vi "MegaAnalysis5.vi"() -> ()   [LabVIEW 2016] (continued)
                          frame #4 {
                            n844 = Array Size(array=w2082) -> (size(s)=w2081:i32)
                            n845 = Divide(x=w2081, y=2) -> (x/y=w2079:dbl)
                            n846 = for {
                              N: w2079 -> [_]
                              tunnel: w2078 -> [w2087]
                              tunnel: w2077 -> [w2084]
                              tunnel: w2076 -> [w2083]
                              i -> [w2088]
                              n847 = Multiply(x=2, y=w2088) -> (x*y=w2091:i32)
                              n848 = Increment(x=w2091) -> (x+1=w2090:i32)
                              n849 = call "readbinary.vi"(7:w2084, "base path"=w2087, "file index"=w2090, "data column"="bdot") -> ("data"=w2086:ext[])  [unwired: 7 out]
                              n850 = call "writebinary.vi"(7:w2083, "base path"=w2087, "file index"=w2088, "data column"="bdtt", "data"=w2086) -> ()  [unwired: 7 out]
                            }
                          }
                          frame #5 {
                            n851 = Array Size(array=w2099) -> (size(s)=w2098:i32)
                            n852 = Divide(x=w2098, y=2) -> (x/y=w2096:dbl)
                            n853 = for {
                              N: w2096 -> [_]
                              tunnel: w2095 -> [w2104]
                              tunnel: w2094 -> [w2101]
                              tunnel: w2093 -> [w2100]
                              i -> [w2105]
                              n854 = Multiply(x=2, y=w2105) -> (x*y=w2107:i32)
                              n855 = Increment(x=w2107) -> ()  [unwired: 1 out]
                              n856 = call "readbinary.vi"(7:w2101, "base path"=w2104, "file index"=w2107, "data column"="indx") -> ("data"=w2103:ext[])  [unwired: 7 out]
                              n857 = call "writebinary.vi"(7:w2100, "base path"=w2104, "file index"=w2105, "data column"="indt", "data"=w2103) -> ()  [unwired: 7 out]
                            }
                          }
                          frame #6 {
                            n858 = Array Size(array=w2115) -> (size(s)=w2114:i32)
                            n859 = Divide(x=w2114, y=2) -> (x/y=w2112:dbl)
                            n860 = for {
                              N: w2112 -> [_]
                              tunnel: w2111 -> [w2120]
                              tunnel: w2110 -> [w2117]
                              tunnel: w2109 -> [w2116]
                              i -> [w2121]
                              n861 = Multiply(x=2, y=w2121) -> (x*y=w2123:i32)
                              n862 = Increment(x=w2123) -> ()  [unwired: 1 out]
                              n863 = call "readbinary.vi"(7:w2117, "base path"=w2120, "file index"=w2123, "data column"="time") -> ("data"=w2119:ext[])  [unwired: 7 out]
                              n864 = call "writebinary.vi"(7:w2116, "base path"=w2120, "file index"=w2121, "data column"="timt", "data"=w2119) -> ()  [unwired: 7 out]
                            }
                          }
                          frame #7 {
                            n865 = Array Size(array=w2136) -> (size(s)=w2139:i32)
                            n866 = Divide(x=w2139, y=2) -> (x/y=w2137:dbl)
                            n867 = for {
                              N: w2137 -> [_]
                              tunnel: w2125 -> [_]
                              tunnel: w2136 -> [w2148]
                              tunnel: w2135 -> [w2147]
                              tunnel: w2134 -> [w2144]
                              tunnel: [w2143] -> w2127 mode=indexing
                              tunnel: w2133 -> [w2142]
                              tunnel: [w2140] -> w2128 mode=indexing
                              i -> [w2150]
                              n868 = Multiply(x=2, y=w2150) -> (x*y=w2141:i32)
                              n869 = Index Array(array=w2148, index=w2141) -> (element=w2146:string)
                              n870 = Increment(x=w2141) -> (x+1=w2149:i32)
                              n871 = Index Array(array=w2148, index=w2149) -> (element=w2145:string)
                              n872 = case shown="1" w2147 {
                                tunnel: w2146 -> [_ w2158]
                                tunnel: w2145 -> [w2152 w2157]
                                tunnel: [w2152 w2155] -> w2143
                                tunnel: w2144 -> [_ w2156]
                                frame 0, Default {
                                }
                                frame 1 {
                                n873 = String Subset(string=w2158, length (rest)=w2156) -> (substring=w2154:string)  [unwired: 1 out]
                                n874 = String Subset(string=w2157, length (rest)=w2156) -> (substring=w2153:string)  [unwired: 1 out]
                                n875 = Concatenate Strings(w2153, w2154) -> (w2155:string)
                                }
                              }
                              n876 = Index Array(array=w2142, index=w2141) -> (element=w2140:path)
                            }
                            n877 = Build Path(base path=w2125, name or relative path="files2") -> (appended path=w2131:path)
                            n878 = call-poly <vilib>:"Write To Spreadsheet File.vi"("1D data"=w2127, "file path (dialog if empty)"=w2131) -> ()  [unwired: 4 in, 3 out]
                            n879 = Build Path(base path=w2125, name or relative path="paths2") -> (appended path=w2129:path)
                            n880 = Path To String(path=w2128) -> (string=w2126:string[])
                            n881 = call-poly <vilib>:"Write To Spreadsheet File.vi"("1D data"=w2126, "file path (dialog if empty)"=w2129) -> ()  [unwired: 4 in, 3 out]
                          }
                        }
                      }
                    }
                  }
                }
                n882 = global write "status.vi" "String"("selecting data") -> ()
              }
            }
          }
          frame #2 {
            n883 = case shown="True" "?" {
              tunnel: w2162 -> [_ w2167]
              tunnel: w2161 -> [_ w2166]
              tunnel: w2160 -> [_ w2165]
              tunnel: w2159 -> [_ w2164]
              frame False {
              }
              frame True {
                n884 = case shown="True" w2165 {
                  tunnel: w2167 -> [_ w2170]
                  tunnel: w2166 -> [_ w2169]
                  tunnel: w2164 -> [_ w2168]
                  frame False {
                  }
                  frame True {
                    n885 = stacked-sequence {
                      seq-local: [w2181 _] -> [_ w2212]
                      seq-local: [w2182 _] -> [_ w2215]
                      seq-local: [w2173 _] -> [_ w2206]
                      seq-local: [w2172 _] -> [_ w2204]
                      tunnel: w2170 -> [w2177 _]
                      tunnel: w2169 -> [w2180 _]
                      tunnel: w2168 -> [w2171 _]
                      frame #0 {
                        n886 = Build Path(base path=w2177, name or relative path="paths2") -> (appended path=w2172:path)
                        n887 = Build Path(base path=w2177, name or relative path="files2") -> (appended path=w2173:path)
                        n888 = call "readbinary.vi"(7:w2171, "base path"=w2177, "file index"=0, "data column"="indt") -> ("data"=w2176:ext[])  [unwired: 7 out]
                        n889 = call-poly <vilib>:"Read From Spreadsheet File.vi"("file path (dialog if empty)"=w2172) -> ("first row"=w2183:string[])  [unwired: 3 in, 7 out]
                        n890 = Array Size(array=w2176) -> (size(s)=w2175:i32)
                        n891 = for {
                          N: w2175 -> [_]
                          tunnel: [0] -> w2174 mode=indexing
                        }
                        n892 = call-poly <vilib>:"Read From Spreadsheet File.vi"("file path (dialog if empty)"=w2173) -> ("first row"=w2181:string[])  [unwired: 3 in, 7 out]
                        n893 = String To Path(string=w2183) -> (path=w2182:path[])
                        n894 = for {
                          tunnel: w2181 -> [w2194]
                          tunnel: w2180 -> [w2191] mode=indexing
                          tunnel: w2177 -> [w2190]
                          tunnel: w2174 -> [w2195]
                          tunnel: w2171 -> [w2187]
                          n895 = Array Size(array=w2194) -> (size(s)=w2189:i32)
                          n896 = for {
                            N: w2189 -> [_]
                            tunnel: w2194 -> [_] mode=indexing
                            tunnel: w2190 -> [w2202]
                            shift-right: [w2201] -> w2193
                            shift-left: w2195 -> [w2199]
                            tunnel: w2191 -> [w2198]
                            tunnel: w2187 -> [w2196]
                            i -> [w2197]
                            n897 = call "readbinary.vi"(7:w2196, "base path"=w2202, "file index"=w2197, "data column"=w2198) -> ("data"=w2200:ext[])  [unwired: 7 out]
                            n898 = Add(x=w2200, y=w2199) -> (x+y=w2201:ext[])
                          }
                          n899 = Divide(x=w2193, y=w2189) -> (x/y=w2192:ext[])
                          n900 = call "writebinary.vi"(7:w2187, "base path"=w2190, "file index"=0, "data column"=w2191, "data"=w2192) -> ()  [unwired: 7 out]
                        }
                      }
                      frame #1 {
                        n901 = Index Array(array=w2215, index=0) -> (element=w2209:path)
                        n902 = case shown="True" "?" {
                          tunnel: w2212 -> [w2219 w2223]
                          tunnel: "append string onto file name" -> [w2218 w2224]
                          tunnel: "?" -> [_ w2222]
                          tunnel: [w2216 w2221] -> w2208
                          frame False {
                            n903 = Index Array(array=w2219, index=0) -> (element=w2217:string)
                            n904 = Concatenate Strings(w2218, w2217) -> (w2216:string)
                          }
                          frame True {
                            n905 = for {
                              shift-right: [w2225] -> w2221
                              shift-left: w2224 -> [w2227]
                              tunnel: w2223 -> [w2230] mode=indexing
                              tunnel: w2222 -> [w2228]
                              n906 = String Subset(string=w2230, offset (0)=0, length (rest)=w2228) -> (substring=w2226:string)
                              n907 = Concatenate Strings(w2227, w2226) -> (w2225:string)
                            }
                          }
                        }
                        n908 = Build Array(w2209) -> (w2207:path[])
                        n909 = Path To String(path=w2207) -> (string=w2203:string[])
                        n910 = Build Array(w2208) -> (w2205:string[])
                        n911 = call-poly <vilib>:"Write To Spreadsheet File.vi"("1D data"=w2205, "file path (dialog if empty)"=w2206) -> ()  [unwired: 4 in, 3 out]
                        n912 = call-poly <vilib>:"Write To Spreadsheet File.vi"("1D data"=w2203, "file path (dialog if empty)"=w2204) -> ()  [unwired: 4 in, 3 out]
                      }
                    }
                  }
                }
              }
            }
          }
          frame #3 {
            n913 = case shown="False" w2233 {
              tunnel: w2232 -> [_ w2235]
              tunnel: w2231 -> [_ w2234]
              frame False {
              }
              frame True {
                n914 = stacked-sequence {
                  seq-local: [w2236 _ _ _ _ _ _] -> [_ w2242 w2300 w2318 w2336 w2354 w2373]
                  tunnel: w2235 -> [w2239 w2243 w2301 w2319 w2337 w2355 w2374]
                  tunnel: [w2236 _ _ _ _ _ _] -> _
                  tunnel: w2234 -> [_ w2241 w2299 w2317 w2335 w2353 w2372]
                  frame #0 {
                    n915 = Build Path(base path=w2239, name or relative path="files2") -> (appended path=w2238:path)
                    n916 = call-poly <vilib>:"Read From Spreadsheet File.vi"("format (%s)"="%s", "file path (dialog if empty)"=w2238) -> ("first row"=w2236:string[])  [unwired: 2 in, 7 out]
                  }
                  frame #1 {
                    n917 = case shown="0, Default" "data options" {
                      tunnel: w2243 -> [w2247 w2256 w2265 w2277 w2289]
                      tunnel: w2242 -> [w2246 w2255 w2264 w2276 w2288]
                      tunnel: w2241 -> [w2245 w2254 w2263 w2275 w2287]
                      frame 0, Default {
                        n918 = for {
                          tunnel: w2247 -> [w2249]
                          tunnel: w2246 -> [_] mode=indexing
                          tunnel: w2245 -> [w2248]
                          i -> [w2250]
                          n919 = call "readbinary.vi"(7:w2248, "base path"=w2249, "file index"=w2250, "data column"="dt1t") -> ("data"=w2252:ext[])  [unwired: 7 out]
                          n920 = call "writebinary.vi"(7:w2248, "base path"=w2249, "file index"=w2250, "data column"="dt1t", "data"=w2252) -> ()  [unwired: 7 out]
                        }
                      }
                      frame 1 {
                        n921 = for {
                          tunnel: w2256 -> [w2258]
                          tunnel: w2255 -> [_] mode=indexing
                          tunnel: w2254 -> [w2257]
                          i -> [w2259]
                          n922 = call "readbinary.vi"(7:w2257, "base path"=w2258, "file index"=w2259, "data column"="dt2t") -> ("data"=w2261:ext[])  [unwired: 7 out]
                          n923 = call "writebinary.vi"(7:w2257, "base path"=w2258, "file index"=w2259, "data column"="dt1t", "data"=w2261) -> ()  [unwired: 7 out]
                        }
                      }
                      frame 2 {
                        n924 = for {
                          tunnel: w2265 -> [w2270]
                          tunnel: w2264 -> [_] mode=indexing
                          tunnel: w2263 -> [w2266]
                          i -> [w2271]
                          n925 = call "readbinary.vi"(7:w2266, "base path"=w2270, "file index"=w2271, "data column"="dt2t") -> ("data"=w2268:ext[])  [unwired: 7 out]
                          n926 = call "readbinary.vi"(7:w2266, "base path"=w2270, "file index"=w2271, "data column"="dt1t") -> ("data"=w2269:ext[])  [unwired: 7 out]
                          n927 = Subtract(x=w2269, y=w2268) -> (x-y=w2267:ext[])
                          n928 = call "writebinary.vi"(7:w2266, "base path"=w2270, "file index"=w2271, "data column"="dt1t", "data"=w2267) -> ()  [unwired: 7 out]
                        }
                      }
                      frame 3 {
                        n929 = for {
                          tunnel: w2277 -> [w2282]
                          tunnel: w2276 -> [_] mode=indexing
                          tunnel: w2275 -> [w2278]
                          i -> [w2283]
                          n930 = call "readbinary.vi"(7:w2278, "base path"=w2282, "file index"=w2283, "data column"="dt2t") -> ("data"=w2280:ext[])  [unwired: 7 out]
                          n931 = call "readbinary.vi"(7:w2278, "base path"=w2282, "file index"=w2283, "data column"="dt1t") -> ("data"=w2281:ext[])  [unwired: 7 out]
                          n932 = Add(x=w2281, y=w2280) -> (x+y=w2279:ext[])
                          n933 = call "writebinary.vi"(7:w2278, "base path"=w2282, "file index"=w2283, "data column"="dt1t", "data"=w2279) -> ()  [unwired: 7 out]
                        }
                      }
                      frame 4 {
                        n934 = for {
                          tunnel: w2289 -> [w2294]
                          tunnel: w2288 -> [_] mode=indexing
                          tunnel: w2287 -> [w2290]
                          i -> [w2295]
                          n935 = call "readbinary.vi"(7:w2290, "base path"=w2294, "file index"=w2295, "data column"="dt2t") -> ("data"=w2292:ext[])  [unwired: 7 out]
                          n936 = call "readbinary.vi"(7:w2290, "base path"=w2294, "file index"=w2295, "data column"="dt1t") -> ("data"=w2293:ext[])  [unwired: 7 out]
                          n937 = Re/Im To Polar(2:w2293, 3:w2292) -> (1:w2291:ext[])  [unwired: 1 out]
                          n938 = call "writebinary.vi"(7:w2290, "base path"=w2294, "file index"=w2295, "data column"="dt1t", "data"=w2291) -> ()  [unwired: 7 out]
                        }
                      }
                    }
                  }
                  frame #2 {
                    n939 = case shown="True" "?" {
                      tunnel: w2301 -> [_ w2305]
                      tunnel: w2300 -> [_ w2304]
                      tunnel: w2299 -> [_ w2303]
                      frame False {
                      }
                      frame True {
                        n940 = for {
                          tunnel: w2305 -> [w2312]
                          tunnel: w2304 -> [_] mode=indexing
                          tunnel: w2303 -> [w2306]
                          i -> [w2313]
                          n941 = call "readbinary.vi"(7:w2306, "base path"=w2312, "file index"=w2313, "data column"="dt1t") -> ("data"=w2308:ext[])  [unwired: 7 out]
                          n942 = call "readbinary.vi"(7:w2306, "base path"=w2312, "file index"=w2313, "data column"="timt") -> ("data"=w2311:ext[])  [unwired: 7 out]
                          n943 = Multiply(x="?", y=w2311) -> (x*y=w2309:ext[])
                          n944 = Add(x=w2308, y=w2309) -> (x+y=w2307:ext[])
                          n945 = call "writebinary.vi"(7:w2306, "base path"=w2312, "file index"=w2313, "data column"="dt1t", "data"=w2307) -> ()  [unwired: 7 out]
                        }
                      }
                    }
                  }
                  frame #3 {
                    n946 = case shown="True" "?" {
                      tunnel: w2319 -> [_ w2323]
                      tunnel: w2318 -> [_ w2322]
                      tunnel: w2317 -> [_ w2321]
                      frame False {
                      }
                      frame True {
                        n947 = for {
                          tunnel: w2323 -> [w2330]
                          tunnel: w2322 -> [_] mode=indexing
                          tunnel: w2321 -> [w2324]
                          i -> [w2331]
                          n948 = call "readbinary.vi"(7:w2324, "base path"=w2330, "file index"=w2331, "data column"="dt1t") -> ("data"=w2326:ext[])  [unwired: 7 out]
                          n949 = call "readbinary.vi"(7:w2324, "base path"=w2330, "file index"=w2331, "data column"="bdtt") -> ("data"=w2329:ext[])  [unwired: 7 out]
                          n950 = Multiply(x="?", y=w2329) -> (x*y=w2327:ext[])
                          n951 = Add(x=w2326, y=w2327) -> (x+y=w2325:ext[])
                          n952 = call "writebinary.vi"(7:w2324, "base path"=w2330, "file index"=w2331, "data column"="dt1t", "data"=w2325) -> ()  [unwired: 7 out]
                        }
                      }
                    }
                  }
                  frame #4 {
                    n953 = case shown="True" "?" {
                      tunnel: w2337 -> [_ w2341]
                      tunnel: w2336 -> [_ w2340]
                      tunnel: w2335 -> [_ w2339]
                      frame False {
                      }
                      frame True {
                        n954 = for {
                          tunnel: w2341 -> [w2348]
                          tunnel: w2340 -> [_] mode=indexing
                          tunnel: w2339 -> [w2342]
                          i -> [w2349]
                          n955 = call "readbinary.vi"(7:w2342, "base path"=w2348, "file index"=w2349, "data column"="dt1t") -> ("data"=w2344:ext[])  [unwired: 7 out]
                          n956 = call "readbinary.vi"(7:w2342, "base path"=w2348, "file index"=w2349, "data column"="bclt") -> ("data"=w2347:ext[])  [unwired: 7 out]
                          n957 = Multiply(x="?", y=w2347) -> (x*y=w2345:ext[])
                          n958 = Add(x=w2344, y=w2345) -> (x+y=w2343:ext[])
                          n959 = call "writebinary.vi"(7:w2342, "base path"=w2348, "file index"=w2349, "data column"="dt1t", "data"=w2343) -> ()  [unwired: 7 out]
                        }
                      }
                    }
                  }
                  frame #5 {
                    n960 = case shown="True" "?" {
                      tunnel: w2355 -> [_ w2359]
                      tunnel: w2354 -> [_ w2358]
                      tunnel: w2353 -> [_ w2357]
                      frame False {
                      }
                      frame True {
                        n961 = for {
                          tunnel: w2359 -> [w2367]
                          tunnel: [w2361] -> _ mode=indexing
                          tunnel: w2358 -> [w2361] mode=indexing
                          tunnel: w2357 -> [w2360]
                          i -> [w2368]
                          n962 = call "readbinary.vi"(7:w2360, "base path"=w2367, "file index"=w2368, "data column"="dt1t") -> ("data"=w2363:ext[])  [unwired: 7 out]
                          n963 = call "readbinary.vi"(7:w2360, "base path"=w2367, "file index"=w2368, "data column"="dt2t") -> ("data"=w2366:ext[])  [unwired: 7 out]
                          n964 = Multiply(x="?", y=w2366) -> (x*y=w2364:ext[])
                          n965 = Add(x=w2363, y=w2364) -> (x+y=w2362:ext[])
                          n966 = call "writebinary.vi"(7:w2360, "base path"=w2367, "file index"=w2368, "data column"="dt1t", "data"=w2362) -> ()  [unwired: 7 out]
                        }
                      }
                    }
                  }
                  frame #6 {
                    n967 = case shown="True" "?" {
                      tunnel: w2374 -> [_ w2378]
                      tunnel: w2373 -> [_ w2377]
                      tunnel: w2372 -> [_ w2376]
                      frame False {
                      }
                      frame True {
                        n968 = for {
                          tunnel: w2378 -> [w2383]
                          tunnel: w2377 -> [_] mode=indexing
                          tunnel: w2376 -> [w2379]
                          i -> [w2384]
                          n969 = call "readbinary.vi"(7:w2379, "base path"=w2383, "file index"=w2384, "data column"="dt1t") -> ("data"=w2381:ext[])  [unwired: 7 out]
                          n970 = Multiply(x="?", y=w2381) -> (x*y=w2380:ext[])
                          n971 = call "writebinary.vi"(7:w2379, "base path"=w2383, "file index"=w2384, "data column"="dt1t", "data"=w2380) -> ()  [unwired: 7 out]
                        }
                      }
                    }
                  }
                }
              }
            }
          }
          frame #4 {
            n972 = case shown="True" w2389 {
              tunnel: w2388 -> [_ w2394]
              tunnel: w2387 -> [_ w2390]
              frame False {
              }
              frame True {
                n973 = Build Path(base path=w2394, name or relative path="files2") -> (appended path=w2392:path)
                n974 = call-poly <vilib>:"Read From Spreadsheet File.vi"("file path (dialog if empty)"=w2392) -> ("first row"=w2391:string[])  [unwired: 3 in, 7 out]
                n975 = for {
                  tunnel: "?" -> [w2399]
                  tunnel: w2394 -> [w2398]
                  tunnel: w2391 -> [_] mode=indexing
                  tunnel: w2390 -> [w2396]
                  i -> [w2397]
                  n976 = case shown="True" w2399 {
                    tunnel: w2398 -> [_ w2407]
                    tunnel: w2397 -> [_ w2406]
                    tunnel: w2396 -> [_ w2400]
                    frame False {
                    }
                    frame True {
                      w2401 = "dt1t"
                      w2402 = "bclt"
                      w2403 = "bdtt"
                      w2404 = "timt"
                      w2405 = "indt"
                      n977 = call "readbinary.vi"(7:w2400, "base path"=w2407, "file index"=w2406, "data column"=w2403) -> ("data"=w2415:ext[])  [unwired: 7 out]
                      n978 = call "readbinary.vi"(7:w2400, "base path"=w2407, "file index"=w2406, "data column"=w2405) -> ("data"=w2417:ext[])  [unwired: 7 out]
                      n979 = call "readbinary.vi"(7:w2400, "base path"=w2407, "file index"=w2406, "data column"=w2404) -> ("data"=w2416:ext[])  [unwired: 7 out]
                      n980 = call "readbinary.vi"(7:w2400, "base path"=w2407, "file index"=w2406, "data column"=w2402) -> ("data"=w2414:ext[])  [unwired: 7 out]
                      n981 = call "readbinary.vi"(7:w2400, "base path"=w2407, "file index"=w2406, "data column"=w2401) -> ("data"=w2413:ext[])  [unwired: 7 out]
                      n982 = call "Btolerance.vi"("index"=w2417, "tolerance (B)"="(slow on large data sets but good for treating small fluctuations in field)", "time"=w2416, "dB/dt"=w2415, "B"=w2414, "data"=w2413) -> ("index 2"=w2412:ext[], "time 2"=w2411:ext[], "dB/dt 2"=w2410:ext[], "B 2"=w2409:ext[], "data 2"=w2408:dbl[])  [unwired: 5 out]
                      n983 = call "writebinary.vi"(7:w2400, "base path"=w2407, "file index"=w2406, "data column"=w2401, "data"=w2408) -> ()  [unwired: 7 out]
                      n984 = call "writebinary.vi"(7:w2400, "base path"=w2407, "file index"=w2406, "data column"=w2404, "data"=w2411) -> ()  [unwired: 7 out]
                      n985 = call "writebinary.vi"(7:w2400, "base path"=w2407, "file index"=w2406, "data column"=w2403, "data"=w2410) -> ()  [unwired: 7 out]
                      n986 = call "writebinary.vi"(7:w2400, "base path"=w2407, "file index"=w2406, "data column"=w2405, "data"=w2412) -> ()  [unwired: 7 out]
                      n987 = call "writebinary.vi"(7:w2400, "base path"=w2407, "file index"=w2406, "data column"=w2402, "data"=w2409) -> ()  [unwired: 7 out]
                    }
                  }
                }
              }
            }
          }
          frame #5 {
            n988 = case shown="False" w2424 {
              tunnel: w2423 -> [_ w2426]
              tunnel: w2422 -> [_ w2429]
              tunnel: w2421 -> [_ w2428]
              tunnel: w2420 -> [_ w2427]
              tunnel: w2419 -> [_ w2425]
              frame False {
              }
              frame True {
                n989 = stacked-sequence {
                  seq-local: [_ w2444 _ _ _ _] -> [_ _ w2484 _ _ _]
                  seq-local: [_ w2446 _ _ _ _] -> [_ _ w2483 _ _ _]
                  seq-local: [_ w2445 _ _ _ _] -> [_ _ w2485 _ _ _]
                  seq-local: [_ _ w2482 _ _ _] -> [_ _ _ _ _ _]
                  seq-local: [_ _ w2481 _ _ _] -> [_ _ _ _ _ _]
                  seq-local: [_ _ w2480 _ _ _] -> [_ _ _ _ w2577 w2614]
                  seq-local: [_ _ w2479 _ _ _] -> [_ _ _ _ w2578 w2615]
                  seq-local: [_ _ _ w2556 _ _] -> [_ _ _ _ _ w2611]
                  seq-local: [_ _ _ w2555 _ _] -> [_ _ _ _ w2576 _]
                  seq-local: [_ _ w2472 _ _ _] -> [_ _ _ _ w2574 w2612]
                  tunnel: w2426 -> [_ w2447 w2475 w2552 w2580 w2616]
                  tunnel: w2429 -> [_ _ _ _ w2581 w2617]
                  tunnel: w2428 -> [_ _ _ _ _ w2610]
                  tunnel: w2427 -> [_ _ _ _ w2579 _]
                  tunnel: w2425 -> [_ w2443 w2474 _ w2575 w2613]
                  frame #0 {
                    n990 = case shown="True" "?" {
                      frame False {
                      }
                      frame True {
                        n991 = property class="XYGraph (strict)"() -> ("CrsrList"=w2436:T17)  [unwired: 2 in, 2 out]
                        n992 = Index Array(array=w2436, index=0) -> (element=w2442:T18)
                        n993 = Index Array(array=w2436, index=1) -> (element=w2439:T18)
                        n994 = Unbundle By Name(w2442) -> ("Position"=w2440:cluster{"X":dbl, "Y":dbl})
                        n995 = Unbundle By Name(w2439) -> ("Position"=w2437:cluster{"X":dbl, "Y":dbl})
                        n996 = Unbundle By Name(w2440) -> ("X"=w2435:dbl)
                        n997 = Unbundle By Name(w2437) -> ("X"=w2434:dbl)
                        n998 = property class="Bool (strict)"("Val(Sgnl)"=TRUE) -> ()  [unwired: 2 in, 2 out]
                        n999 = Bundle("X"=w2435, "X"=w2434) -> (w2433:cluster{"X":dbl, "X":dbl})  [unwired: 1 out]
                        n1000 = Build Array(w2433) -> (w2431:cluster{"X":dbl, "X":dbl}[])
                        n1001 = property class="Arr (strict)"("Val(Sgnl)"=w2431) -> ()  [unwired: 2 in, 2 out]
                      }
                    }
                  }
                  frame #1 {
                    n1002 = Build Path(base path=w2447, name or relative path="files2") -> (appended path=w2448:path)
                    n1003 = call-poly <vilib>:"Read From Spreadsheet File.vi"("file path (dialog if empty)"=w2448) -> ("first row"=w2445:string[])  [unwired: 3 in, 7 out]
                    n1004 = for {
                      tunnel: w2445 -> [_] mode=indexing
                      tunnel: w2447 -> [w2469]
                      tunnel: [w2460] -> w2444 mode=indexing
                      tunnel: [w2459] -> w2446 mode=indexing
                      tunnel: w2443 -> [w2452]
                      i -> [w2470]
                      (unwired) inf
                      (unwired) -inf
                      w2464 = 0
                      n1005 = call "readbinary.vi"(7:w2452, "base path"=w2469, "file index"=w2470, "data column"="bclt") -> ("data"=w2467:ext[])  [unwired: 7 out]
                      n1006 = Array Size(array=w2467) -> (size(s)=w2454:i32)
                      n1007 = Less?(x="threshold # of points below which field variations are ignored", y=w2454) -> (x < y?=w2456:bool)
                      n1008 = Select(t="threshold # of points below which field variations are ignored", s=w2456, f=w2454) -> (s? t:f=w2453:dbl)
                      n1009 = Decrement(x=w2454) -> (x-1=w2465:i32)
                      n1010 = call-poly <vilib>:"Waveform Peak Detection.vi"("width"=w2453, "threshold"="maxima above:", "Signal In"=w2467) -> ("Amplitudes"=w2462:dbl[], "Locations"=w2466:dbl[])  [unwired: 4 in, 3 out]
                      n1011 = call-poly <vilib>:"Waveform Peak Detection.vi"("peaks/valleys"=1, "width"=w2453, "threshold"="minima below :", "Signal In"=w2467) -> ("Amplitudes"=w2458:dbl[], "Locations"=w2457:dbl[])  [unwired: 3 in, 3 out]
                      n1012 = Index Array(array=w2467, index=w2464) -> (element=w2463:ext)
                      n1013 = Index Array(array=w2467, index=w2465) -> (element=w2461:ext)
                      n1014 = Build Array (concatenate)(w2464, w2466, w2457, w2465) -> (w2460:dbl[])
                      n1015 = Build Array (concatenate)(w2463, w2462, w2458, w2461) -> (w2459:ext[])
                    }
                  }
                  frame #2 {
                    n1016 = for {
                      tunnel: w2485 -> [_] mode=indexing
                      tunnel: w2484 -> [w2507] mode=indexing
                      tunnel: w2483 -> [w2506] mode=indexing
                      tunnel: [w2502] -> w2482 mode=indexing
                      tunnel: [w2501] -> w2481 mode=indexing
                      tunnel: [w2500] -> w2480 mode=indexing
                      tunnel: [w2499] -> w2479 mode=indexing
                      tunnel: [w2490] -> w2477 mode=indexing
                      tunnel: w2475 -> [w2498]
                      tunnel: [w2495] -> w2473 mode=indexing
                      tunnel: w2474 -> [w2493]
                      tunnel: [w2491] -> w2472 mode=indexing
                      i -> [w2497]
                      w2503 = dbl[] [] ("Array 10")
                      n1017 = Array Size(array=w2506) -> (size(s)=w2505:i32)
                      n1018 = for {
                        N: w2505 -> [_]
                        shift-right: [w2545] -> _
                        shift-left: w2507 -> [w2548]
                        tunnel: [w2550] -> w2488 mode=indexing
                        tunnel: [w2549] -> w2489 mode=indexing
                        tunnel: w2506 -> [w2544]
                        n1019 = Array Max & Min(array=w2548) -> (min value=w2550:dbl, min index (indices)=w2547:i32)  [unwired: 2 out]
                        n1020 = Index Array(array=w2544, index=w2547) -> (element=w2549:ext)
                        n1021 = Replace Array Subset(array=w2548, new element=inf, index=w2547) -> (w2545:dbl[])
                      }
                      n1022 = call "removezeroes.vi"("index"=w2488, "B"=w2489) -> ("index out"=w2486:dbl[], "B out"=w2487:dbl[])  [unwired: 8 out]
                      n1023 = call "Btolerance.vi"("tolerance (B)"="consider variations in B field only above:", "B"=w2487, "data"=w2486) -> ("B 2"=w2490:ext[], "data 2"=w2491:dbl[])  [unwired: 3 in, 8 out]
                      n1024 = Decrement(x=w2505) -> (x-1=w2504:i32)
                      n1025 = for {
                        N: w2504 -> [_]
                        tunnel: w2491 -> [w2523]
                        tunnel: w2490 -> [w2527]
                        shift-right: [w2516] -> w2502
                        shift-left: w2503 -> [w2518]
                        shift-right: [w2515] -> w2501
                        shift-left: w2503 -> [w2517]
                        shift-right: [w2514] -> w2500
                        shift-left: w2503 -> [w2512]
                        shift-right: [w2513] -> w2499
                        shift-left: w2503 -> [w2511]
                        i -> [w2521]
                        n1026 = Increment(x=w2521) -> (x+1=w2522:i32)
                        n1027 = Index Array(array=w2527, index=w2522) -> (element=w2526:ext)
                        n1028 = Index Array(array=w2527, index=w2521) -> (element=w2525:ext)
                        n1029 = Index Array(array=w2523, index=w2522) -> (element=w2519:dbl)
                        n1030 = Index Array(array=w2523, index=w2521) -> (element=w2520:dbl)
                        n1031 = Greater?(x=w2526, y=w2525) -> (0:w2524:bool)
                        n1032 = case shown="True" w2524 {
                          tunnel: w2520 -> [w2529 w2540]
                          tunnel: w2519 -> [w2528 w2541]
                          tunnel: w2518 -> [w2535 w2543]
                          tunnel: w2517 -> [w2534 w2542]
                          tunnel: [w2535 w2539] -> w2516
                          tunnel: [w2534 w2538] -> w2515
                          tunnel: [w2533 w2537] -> w2514
                          tunnel: [w2532 w2536] -> w2513
                          tunnel: w2512 -> [w2531 w2537]
                          tunnel: w2511 -> [w2530 w2536]
                          frame False {
                            n1033 = Build Array (concatenate)(w2531, w2529) -> (w2533:dbl[])
                            n1034 = Build Array (concatenate)(w2530, w2528) -> (w2532:dbl[])
                          }
                          frame True {
                            n1035 = Build Array (concatenate)(w2543, w2540) -> (w2539:dbl[])
                            n1036 = Build Array (concatenate)(w2542, w2541) -> (w2538:dbl[])
                          }
                        }
                      }
                      n1037 = call "readbinary.vi"(7:w2493, "base path"=w2498, "file index"=w2497, "data column"="indt") -> ("data"=w2492:ext[])  [unwired: 7 out]
                      n1038 = for {
                        tunnel: w2492 -> [w2510]
                        tunnel: w2491 -> [w2509] mode=indexing
                        tunnel: [w2508] -> w2495 mode=indexing
                        n1039 = Index Array(array=w2510, index=w2509) -> (element=w2508:ext)
                      }
                    }
                    n1040 = Transpose 2D Array(2D array=w2473) -> (transposed array=→"row":ext[][])
                    n1041 = Transpose 2D Array(2D array=w2477) -> (transposed array=→"fields":ext[][])
                  }
                  frame #3 {
                    n1042 = Build Path(base path=w2552, name or relative path="files2") -> (appended path=w2553:path)
                    n1043 = call-poly <vilib>:"Read From Spreadsheet File.vi"("file path (dialog if empty)"=w2553) -> ("first row"=w2551:string[])  [unwired: 3 in, 7 out]
                    n1044 = case shown="True" "?" {
                      tunnel: "falling sweep start index" -> [w2560 w2568]
                      tunnel: "rising sweep start index" -> [w2561 w2567]
                      tunnel: [w2561 w2563] -> w2556
                      tunnel: [w2560 w2562] -> w2555
                      tunnel: w2551 -> [_ w2571]
                      frame False {
                      }
                      frame True {
                        n1045 = Array Size(array=w2571) -> (size(s)=w2566:i32)
                        n1046 = Index Array(array=w2568, index=0) -> (element=w2565:dbl)
                        n1047 = Index Array(array=w2567, index=0) -> (element=w2564:dbl)
                        n1048 = for {
                          N: w2566 -> [_]
                          tunnel: [w2573] -> w2563 mode=indexing
                          tunnel: w2564 -> [w2573]
                        }
                        n1049 = for {
                          N: w2566 -> [_]
                          tunnel: w2565 -> [w2572]
                          tunnel: [w2572] -> w2562 mode=indexing
                        }
                      }
                    }
                  }
                  frame #4 {
                    n1050 = for {
                      tunnel: w2577 -> [w2596] mode=indexing
                      tunnel: w2578 -> [w2595] mode=indexing
                      tunnel: w2576 -> [w2594] mode=indexing
                      tunnel: w2576 -> [w2588] mode=indexing
                      tunnel: w2581 -> [w2593]
                      tunnel: w2579 -> [w2592]
                      tunnel: w2580 -> [w2591]
                      tunnel: w2575 -> [w2589]
                      tunnel: w2574 -> [w2586] mode=indexing
                      tunnel: [w2583] -> _ mode=indexing
                      tunnel: [w2582] -> _ mode=indexing
                      i -> [w2590]
                      n1051 = Increment(x=w2588) -> (x+1=w2587:dbl)
                      n1052 = Index Array(array=w2596, index=w2594) -> ()  [unwired: 1 out]
                      n1053 = Index Array(array=w2595, index=w2588) -> ()  [unwired: 1 out]
                      n1054 = Index Array(array=w2586, index=w2588) -> (element=w2584:dbl)
                      n1055 = Index Array(array=w2586, index=w2587) -> (element=w2585:dbl)
                      n1056 = for {
                        tunnel: w2593 -> [w2605] mode=indexing
                        tunnel: w2592 -> [w2602] mode=indexing
                        tunnel: w2584 -> [w2607]
                        tunnel: w2585 -> [w2609]
                        tunnel: w2591 -> [w2603]
                        tunnel: w2590 -> [w2604]
                        tunnel: w2589 -> [w2601]
                        tunnel: [w2599] -> w2583 mode=indexing
                        tunnel: [w2597] -> w2582 mode=indexing
                        n1057 = Subtract(x=w2609, y=w2607) -> (x-y=w2608:dbl)
                        n1058 = call "readbinary.vi"(7:w2601, "base path"=w2603, "file index"=w2604, "data column"=w2605) -> ("data"=w2598:ext[])  [unwired: 7 out]
                        n1059 = Increment(x=w2608) -> (x+1=w2606:dbl)
                        n1060 = Array Subset(array=w2598, index=w2607, length=w2606) -> (w2600:ext[])
                        n1061 = Array Size(array=w2598) -> (size(s)=w2597:i32)
                        n1062 = call "writebinary.vi"(7:w2601, "base path"=w2603, "file index"=w2604, "data column"=w2602, "data"=w2600) -> ()  [unwired: 7 out]
                        n1063 = Array Size(array=w2600) -> (size(s)=w2599:i32)
                      }
                    }
                  }
                  frame #5 {
                    n1064 = for {
                      tunnel: w2614 -> [w2632] mode=indexing
                      tunnel: w2615 -> [w2631] mode=indexing
                      tunnel: w2611 -> [w2630] mode=indexing
                      tunnel: w2611 -> [w2624] mode=indexing
                      tunnel: w2617 -> [w2629]
                      tunnel: w2610 -> [w2628]
                      tunnel: w2616 -> [w2627]
                      tunnel: w2613 -> [w2625]
                      tunnel: w2612 -> [w2622] mode=indexing
                      tunnel: [w2619] -> _ mode=indexing
                      tunnel: [w2618] -> _ mode=indexing
                      i -> [w2626]
                      n1065 = Increment(x=w2624) -> (x+1=w2623:dbl)
                      n1066 = Index Array(array=w2632, index=w2630) -> ()  [unwired: 1 out]
                      n1067 = Index Array(array=w2631, index=w2624) -> ()  [unwired: 1 out]
                      n1068 = Index Array(array=w2622, index=w2624) -> (element=w2620:dbl)
                      n1069 = Index Array(array=w2622, index=w2623) -> (element=w2621:dbl)
                      n1070 = for {
                        tunnel: w2629 -> [w2641] mode=indexing
                        tunnel: w2628 -> [w2638] mode=indexing
                        tunnel: w2620 -> [w2643]
                        tunnel: w2621 -> [w2645]
                        tunnel: w2627 -> [w2639]
                        tunnel: w2626 -> [w2640]
                        tunnel: w2625 -> [w2637]
                        tunnel: [w2635] -> w2619 mode=indexing
                        tunnel: [w2633] -> w2618 mode=indexing
                        n1071 = Subtract(x=w2645, y=w2643) -> (x-y=w2644:dbl)
                        n1072 = call "readbinary.vi"(7:w2637, "base path"=w2639, "file index"=w2640, "data column"=w2641) -> ("data"=w2634:ext[])  [unwired: 7 out]
                        n1073 = Increment(x=w2644) -> (x+1=w2642:dbl)
                        n1074 = Array Subset(array=w2634, index=w2643, length=w2642) -> (w2636:ext[])
                        n1075 = Array Size(array=w2634) -> (size(s)=w2633:i32)
                        n1076 = call "writebinary.vi"(7:w2637, "base path"=w2639, "file index"=w2640, "data column"=w2638, "data"=w2636) -> ()  [unwired: 7 out]
                        n1077 = Array Size(array=w2636) -> (size(s)=w2635:i32)
                      }
                    }
                  }
                }
              }
            }
          }
          frame #6 {
            n1078 = Not Equal To 0?(x="field limits:") -> (x != 0?=w2647:bool)
            n1079 = case shown="True" w2654 {
              tunnel: w2647 -> [_ w2666]
              tunnel: w2653 -> [_ w2665]
              tunnel: w2652 -> [_ w2664]
              tunnel: w2651 -> [_ w2663]
              tunnel: w2650 -> [_ w2662]
              tunnel: "field smoothing" -> [_ w2661]
              tunnel: "offset options" -> [_ w2660]
              tunnel: "field limits:" -> [_ w2656]
              frame False {
              }
              frame True {
                n1080 = case shown="False" w2666 {
                  tunnel: w2665 -> [_ w2685]
                  tunnel: w2664 -> [_ w2684]
                  tunnel: w2663 -> [_ w2683]
                  tunnel: w2662 -> [_ w2682]
                  tunnel: w2661 -> [_ w2680]
                  tunnel: "smoothing ratio (must be appreciably larger than 1)" -> [_ w2679]
                  tunnel: w2660 -> [_ w2678]
                  tunnel: "offset value" -> [_ w2677]
                  tunnel: "sweeprate-dependent  offset multiplier" -> [_ w2676]
                  tunnel: w2656 -> [_ w2670]
                  tunnel: "field margin for interpolation" -> [_ w2675]
                  frame False {
                  }
                  frame True {
                    n1081 = Build Path(base path=w2685, name or relative path="files2") -> (appended path=w2687:path)
                    n1082 = call-poly <vilib>:"Read From Spreadsheet File.vi"("file path (dialog if empty)"=w2687) -> ("first row"=w2686:string[])  [unwired: 3 in, 7 out]
                    n1083 = Equal?(x=w2670, y=2) -> (x = y?=w2668:bool)
                    n1084 = for {
                      tunnel: w2686 -> [w2696] mode=indexing
                      tunnel: w2685 -> [w2702]
                      tunnel: w2684 -> [w2701]
                      tunnel: w2683 -> [w2700]
                      tunnel: w2682 -> [w2699]
                      tunnel: "?" -> [w2698]
                      tunnel: w2680 -> [w2697]
                      tunnel: w2679 -> [w2695]
                      tunnel: w2678 -> [w2694]
                      tunnel: w2677 -> [w2693]
                      tunnel: w2676 -> [w2692]
                      tunnel: w2670 -> [w2691]
                      tunnel: w2675 -> [w2690]
                      tunnel: [w2689] -> w2674 mode=indexing
                      i -> [w2703]
                      n1085 = stacked-sequence {
                        seq-local: [_ w2730 _ _ _ _ _ _ _ _] -> [_ _ _ _ w2777 _ _ _ _ _]
                        seq-local: [_ w2729 _ _ _ _ _ _ _ _] -> [_ _ _ _ w2776 _ _ _ _ _]
                        seq-local: [_ _ w2746 _ _ _ _ _ _ _] -> [_ _ _ _ _ w2797 _ _ _ _]
                        seq-local: [_ _ w2745 _ _ _ _ _ _ _] -> [_ _ _ _ _ w2796 _ _ _ _]
                        seq-local: [w2709 _ _ _ _ _ _ _ _ _] -> [_ w2732 w2748 _ _ _ _ _ _ _]
                        seq-local: [w2708 _ _ _ _ _ _ _ _ _] -> [_ w2731 w2747 _ _ _ _ _ _ _]
                        seq-local: [_ _ _ _ _ _ _ _ w2919 _] -> [_ _ _ _ _ _ _ _ _ w2995]
                        seq-local: [_ _ _ _ _ _ _ _ w2918 _] -> [_ _ _ _ _ _ _ _ _ w2993]
                        seq-local: [_ _ _ _ _ _ _ _ w2917 _] -> [_ _ _ _ _ _ _ _ _ w2994]
                        seq-local: [_ _ _ _ _ _ _ _ w2916 _] -> [_ _ _ _ _ _ _ _ _ w2992]
                        seq-local: [w2705 _ _ _ _ _ _ _ _ _] -> [_ _ _ w2768 _ _ _ _ _ _]
                        seq-local: [w2704 _ _ _ _ _ _ _ _ _] -> [_ _ _ w2767 _ _ _ _ _ _]
                        seq-local: [_ _ w2744 _ _ _ _ _ _ _] -> [_ _ _ w2774 _ _ _ _ _ _]
                        seq-local: [_ w2728 _ _ _ _ _ _ _ _] -> [_ _ _ w2773 _ _ _ _ _ _]
                        tunnel: w2703 -> [w2715 w2742 w2758 _ w2779 w2800 w2816 w2855 w2921 w2998]
                        tunnel: w2702 -> [_ w2741 w2757 _ w2778 w2799 w2819 w2856 w2920 w2997]
                        tunnel: w2701 -> [_ _ _ _ w2780 _ _ _ _ w3000]
                        tunnel: w2700 -> [_ _ _ _ _ w2798 _ _ _ w2999]
                        tunnel: w2699 -> [_ w2733 w2749 _ w2775 w2795 w2818 w2854 w2922 w2996]
                        tunnel: w2698 -> [w2714 _ _ _ _ _ _ _ _ _]
                        tunnel: w2697 -> [_ _ _ _ _ _ w2820 _ _ _]
                        tunnel: w2696 -> [_ _ _ _ _ _ w2817 _ _ _]
                        tunnel: w2695 -> [_ _ _ _ _ _ w2815 _ _ _]
                        tunnel: w2694 -> [_ _ _ _ _ _ _ w2857 w2923 w3001]
                        tunnel: w2693 -> [_ _ _ _ _ _ _ w2853 _ _]
                        tunnel: w2692 -> [_ _ _ _ _ _ _ w2852 _ _]
                        tunnel: w2691 -> [w2710 _ _ _ _ _ _ _ _ _]
                        tunnel: w2690 -> [w2706 _ _ _ _ _ _ _ _ _]
                        tunnel: [_ _ _ w2762 _ _ _ _ _ _] -> w2689
                        frame #0 {
                          n1086 = Equal?(x=w2710, y=2) -> (x = y?=w2707:bool)
                          n1087 = case shown="False" "?" {
                            tunnel: [w2726 0] -> w2713
                            tunnel: w2715 -> [w2726 _]
                            frame False {
                            }
                            frame True {
                            }
                          }
                          n1088 = Index Array(array=w2714, index=w2713) -> (element=w2712:cluster{dbl, "and":dbl})
                          n1089 = Unbundle(w2712) -> (w2705:dbl, "and"=w2704:dbl)
                          n1090 = case shown="False" w2707 {
                            tunnel: w2705 -> [w2719 w2725]
                            tunnel: [w2719 w2723] -> w2709
                            tunnel: w2704 -> [w2718 w2724]
                            tunnel: [w2718 w2722] -> w2708
                            tunnel: w2706 -> [_ w2721]
                            frame False {
                              n1091 = property class="Bool (strict)"("Val(Sgnl)"=TRUE) -> ()  [unwired: 2 in, 2 out]
                            }
                            frame True {
                              n1092 = Subtract(x=w2725, y=w2721) -> (x-y=w2723:dbl)
                              n1093 = Add(x=w2724, y=w2721) -> (x+y=w2722:dbl)
                              n1094 = property class="Bool (strict)"("Val(Sgnl)"=FALSE) -> ()  [unwired: 2 in, 2 out]
                            }
                          }
                        }
                        frame #1 {
                          n1095 = call "readbinary.vi"(7:w2733, "base path"=w2741, "file index"=w2742, "data column"="bclr") -> ("data"=w2728:ext[])  [unwired: 7 out]
                          n1096 = Subtract(x=w2728, y=w2731) -> (x-y=w2738:ext[])
                          n1097 = Subtract(x=w2728, y=w2732) -> (x-y=w2740:ext[])
                          n1098 = Absolute Value(x=w2738) -> (abs(x)=w2737:ext[])
                          n1099 = Absolute Value(x=w2740) -> (abs(x)=w2739:ext[])
                          n1100 = Array Max & Min(array=w2737) -> (min index (indices)=w2735:i32)  [unwired: 3 out]
                          n1101 = Array Max & Min(array=w2739) -> (min index (indices)=w2736:i32)  [unwired: 3 out]
                          n1102 = Build Array(w2736, w2735) -> (w2734:i32[])
                          n1103 = Array Max & Min(array=w2734) -> (max value=w2729:i32, min value=w2730:i32)  [unwired: 2 out]
                        }
                        frame #2 {
                          n1104 = call "readbinary.vi"(7:w2749, "base path"=w2757, "file index"=w2758, "data column"="bclf") -> ("data"=w2744:ext[])  [unwired: 7 out]
                          n1105 = Subtract(x=w2744, y=w2747) -> (x-y=w2754:ext[])
                          n1106 = Subtract(x=w2744, y=w2748) -> (x-y=w2756:ext[])
                          n1107 = Absolute Value(x=w2754) -> (abs(x)=w2753:ext[])
                          n1108 = Absolute Value(x=w2756) -> (abs(x)=w2755:ext[])
                          n1109 = Array Max & Min(array=w2753) -> (min index (indices)=w2751:i32)  [unwired: 3 out]
                          n1110 = Array Max & Min(array=w2755) -> (min index (indices)=w2752:i32)  [unwired: 3 out]
                          n1111 = Build Array(w2752, w2751) -> (w2750:i32[])
                          n1112 = Array Max & Min(array=w2750) -> (max value=w2745:i32, min value=w2746:i32)  [unwired: 2 out]
                        }
                        frame #3 {
                          n1113 = Array Max & Min(array=w2774) -> (max value=w2772:ext, min value=w2770:ext)  [unwired: 2 out]
                          n1114 = Array Max & Min(array=w2773) -> (max value=w2771:ext, min value=w2769:ext)  [unwired: 2 out]
                          n1115 = Max & Min(x=w2772, y=w2771) -> (min(x,y)=w2765:ext)  [unwired: 1 out]
                          n1116 = Max & Min(x=w2770, y=w2769) -> (max(x,y)=w2761:ext)  [unwired: 1 out]
                          n1117 = Max & Min(x=w2768, y=w2767) -> (max(x,y)=w2766:dbl, min(x,y)=w2760:dbl)
                          n1118 = Greater?(x=w2766, y=w2765) -> (0:w2764:bool)
                          n1119 = Less?(x=w2760, y=w2761) -> (x < y?=w2763:bool)
                          n1120 = Or(x=w2764, y=w2763) -> (x .or. y?=w2762:bool)
                        }
                        frame #4 {
                          n1121 = for {
                            tunnel: w2780 -> [w2788] mode=indexing
                            tunnel: w2779 -> [w2787]
                            tunnel: w2778 -> [w2786]
                            tunnel: w2777 -> [w2790]
                            tunnel: w2776 -> [w2789]
                            tunnel: w2775 -> [w2785]
                            n1122 = call "readbinary.vi"(7:w2785, "base path"=w2786, "file index"=w2787, "data column"=w2788) -> ("data"=w2791:ext[])  [unwired: 7 out]
                            n1123 = Subtract(x=w2789, y=w2790) -> (x-y=w2782:i32)
                            n1124 = Greater Than 0?(x=w2782) -> (x > 0?=w2783:bool)
                            n1125 = case shown="True" w2783 {
                              tunnel: w2782 -> [_ w2794]
                              tunnel: [0 w2793] -> w2781
                              frame False {
                              }
                              frame True {
                                n1126 = Increment(x=w2794) -> (x+1=w2793:i32)
                              }
                            }
                            n1127 = Array Subset(array=w2791, index=w2790, length=w2781) -> (w2784:ext[])
                            n1128 = call "writebinary.vi"(7:w2785, "base path"=w2786, "file index"=w2787, "data column"=w2788, "data"=w2784) -> ()  [unwired: 7 out]
                          }
                        }
                        frame #5 {
                          n1129 = for {
                            tunnel: w2798 -> [w2808] mode=indexing
                            tunnel: w2800 -> [w2807]
                            tunnel: w2799 -> [w2806]
                            tunnel: w2797 -> [w2810]
                            tunnel: w2796 -> [w2809]
                            tunnel: w2795 -> [w2805]
                            n1130 = call "readbinary.vi"(7:w2805, "base path"=w2806, "file index"=w2807, "data column"=w2808) -> ("data"=w2811:ext[])  [unwired: 7 out]
                            n1131 = Subtract(x=w2809, y=w2810) -> (x-y=w2802:i32)
                            n1132 = Greater Than 0?(x=w2802) -> (x > 0?=w2803:bool)
                            n1133 = case shown="True" w2803 {
                              tunnel: w2802 -> [_ w2814]
                              tunnel: [0 w2813] -> w2801
                              frame False {
                              }
                              frame True {
                                n1134 = Increment(x=w2814) -> (x+1=w2813:i32)
                              }
                            }
                            n1135 = Array Subset(array=w2811, index=w2810, length=w2801) -> (w2804:ext[])
                            n1136 = call "writebinary.vi"(7:w2805, "base path"=w2806, "file index"=w2807, "data column"=w2808, "data"=w2804) -> ()  [unwired: 7 out]
                          }
                        }
                        frame #6 {
                          n1137 = case shown="1" w2820 {
                            tunnel: w2819 -> [_ w2825]
                            tunnel: w2818 -> [_ w2826]
                            tunnel: w2817 -> [_ _]
                            tunnel: w2816 -> [_ w2827]
                            tunnel: w2815 -> [_ w2821]
                            frame 0, Default {
                            }
                            frame 1 {
                              n1138 = Build Array("bclr", "bclf") -> (w2822:string[])
                              n1139 = for {
                                tunnel: w2827 -> [w2847]
                                tunnel: w2826 -> [w2846]
                                tunnel: w2825 -> [w2845]
                                tunnel: w2822 -> [w2844] mode=indexing
                                tunnel: w2821 -> [w2843]
                                n1140 = call "readbinary.vi"(7:w2846, "base path"=w2845, "file index"=w2847, "data column"=w2844) -> ("data"=w2834:ext[])  [unwired: 7 out]
                                n1141 = Array Size(array=w2834) -> (size(s)=w2841:i32)
                                n1142 = Divide(x=w2841, y=w2843) -> (x/y=w2842:dbl)
                                n1143 = Round To Nearest(number=w2842) -> (nearest integer value=w2840:dbl)
                                n1144 = Decrement(x=w2841) -> (x-1=w2839:i32)
                                n1145 = for {
                                N: w2840 -> [w2848]
                                tunnel: [w2849] -> w2836 mode=indexing
                                tunnel: [w2848] -> _ mode=indexing
                                i -> [w2849]
                                }
                                n1146 = Decrement(x=w2840) -> (x-1=w2837:dbl)
                                n1147 = for {
                                N: w2841 -> [w2850]
                                tunnel: [w2851] -> w2830 mode=indexing
                                tunnel: [w2850] -> _ mode=indexing
                                i -> [w2851]
                                }
                                n1148 = Multiply(x=w2839, y=w2836) -> (x*y=w2838:i32[])
                                n1149 = call <vilib>:"Linear Fit.vi"("Y"=w2834, "X"=w2830) -> ()  [unwired: 4 in, 10 out]
                                n1150 = Divide(x=w2838, y=w2837) -> (x/y=w2835:dbl[])
                                n1151 = call <vilib>:"Interpolate 1D.vi"("method"=1, "xi"=w2835, "X"=w2830, "Y"=w2834) -> ("xi used"=w2831:dbl[], "yi"=w2832:dbl[])  [unwired: 2 in, 4 out]
                                n1152 = call <vilib>:"Interpolate 1D.vi"("method"=2, "xi"=w2830, "X"=w2831, "Y"=w2832) -> ("yi"=w2828:dbl[])  [unwired: 2 in, 5 out]
                                n1153 = call "writebinary.vi"(7:w2846, "base path"=w2845, "file index"=w2847, "data column"=w2844, "data"=w2828) -> ()  [unwired: 7 out]
                              }
                            }
                          }
                        }
                        frame #7 {
                          n1154 = case shown="0, Default" w2857 {
                            tunnel: w2856 -> [_ w2861 w2878 w2901]
                            tunnel: w2855 -> [_ w2860 w2877 w2900]
                            tunnel: w2854 -> [_ w2859 w2876 w2899]
                            tunnel: w2853 -> [_ w2858 w2875 w2898]
                            tunnel: w2852 -> [_ _ _ w2891]
                            frame 0, Default {
                            }
                            frame 1 {
                              n1155 = Build Array("bclr", "bclf") -> (w2862:string[])
                              n1156 = for {
                                tunnel: w2862 -> [w2867] mode=indexing
                                tunnel: w2861 -> [w2865]
                                tunnel: w2860 -> [w2866]
                                tunnel: w2859 -> [w2868]
                                tunnel: w2858 -> [w2870]
                                n1157 = call "readbinary.vi"(7:w2868, "base path"=w2865, "file index"=w2866, "data column"=w2867) -> ("data"=w2871:ext[])  [unwired: 7 out]
                                n1158 = Add(x=w2871, y=w2870) -> (x+y=w2869:ext[])
                                n1159 = call "writebinary.vi"(7:w2868, "base path"=w2865, "file index"=w2866, "data column"=w2867, "data"=w2869) -> ()  [unwired: 7 out]
                              }
                            }
                            frame 2 {
                              n1160 = Build Array("bclr", "bclf") -> (w2879:string[])
                              n1161 = Build Array(1, -1) -> (w2872:i32[])
                              n1162 = for {
                                tunnel: w2879 -> [w2887] mode=indexing
                                tunnel: w2878 -> [w2885]
                                tunnel: w2877 -> [w2886]
                                tunnel: w2876 -> [w2888]
                                tunnel: w2875 -> [w2884]
                                tunnel: w2872 -> [w2883] mode=indexing
                                n1163 = call "readbinary.vi"(7:w2888, "base path"=w2885, "file index"=w2886, "data column"=w2887) -> ("data"=w2890:ext[])  [unwired: 7 out]
                                n1164 = Multiply(x=w2884, y=w2883) -> (x*y=w2882:dbl)
                                n1165 = Add(x=w2890, y=w2882) -> (x+y=w2889:ext[])
                                n1166 = call "writebinary.vi"(7:w2888, "base path"=w2885, "file index"=w2886, "data column"=w2887, "data"=w2889) -> ()  [unwired: 7 out]
                              }
                            }
                            frame 3 {
                              n1167 = Build Array("bclr", "bclf") -> (w2902:string[])
                              n1168 = Build Array(1, -1) -> (w2895:i32[])
                              n1169 = Build Array("bdtr", "bdtf") -> (w2892:string[])
                              n1170 = for {
                                tunnel: w2902 -> [w2913] mode=indexing
                                tunnel: w2901 -> [w2910]
                                tunnel: w2900 -> [w2911]
                                tunnel: w2899 -> [w2909]
                                tunnel: w2898 -> [_]
                                tunnel: w2895 -> [_] mode=indexing
                                tunnel: w2892 -> [w2912] mode=indexing
                                tunnel: w2891 -> [w2906]
                                n1171 = call "readbinary.vi"(7:w2909, "base path"=w2910, "file index"=w2911, "data column"=w2913) -> ("data"=w2915:ext[])  [unwired: 7 out]
                                n1172 = call "readbinary.vi"(7:w2909, "base path"=w2910, "file index"=w2911, "data column"=w2912) -> ("data"=w2908:ext[])  [unwired: 7 out]
                                n1173 = call-poly <vilib>:"Mean.vi"("X"=w2908) -> ("mean"=w2907:dbl)  [unwired: 1 out]
                                n1174 = Multiply(x=w2907, y=w2906) -> (x*y=w2905:dbl)
                                n1175 = Add(x=w2915, y=w2905) -> (x+y=w2914:ext[])
                                n1176 = call "writebinary.vi"(7:w2909, "base path"=w2910, "file index"=w2911, "data column"=w2913, "data"=w2914) -> ()  [unwired: 7 out]
                              }
                            }
                          }
                        }
                        frame #8 {
                          n1177 = case shown="0, Default" w2923 {
                            tunnel: w2922 -> [_ _ w2956 w2989]
                            tunnel: w2921 -> [_ _ w2955 w2988]
